vi "TestExecuteValueChangeSubscription_RejectRepeats.vi"(8 "error in (no error)":errorcluster, 11 "TestCase in":refnum<class "TestSubscriptionPolicy.lvclass">) -> (0 "error out":errorcluster, 3 "TestCase out":refnum<class "TestSubscriptionPolicy.lvclass">)   [LabVIEW 2015, in "TestSubscriptionPolicy.lvclass"]
uses:
  TestSubscriptionPolicy.lvclass
  Framework/SubscriptionPolicy/ValueChangeSubscription/ValueChangeSubscription.lvclass/ValueChangeSubscription.ctl
  Framework/SubscriptionPolicy/ValueChangeSubscription/ValueChangeSubscription.lvclass
  Framework/Transport/QueueTransport/QueueTransport.lvclass
  Framework/IMediator/ISubscriptionPolicy/ISubscriptionPolicy.lvclass
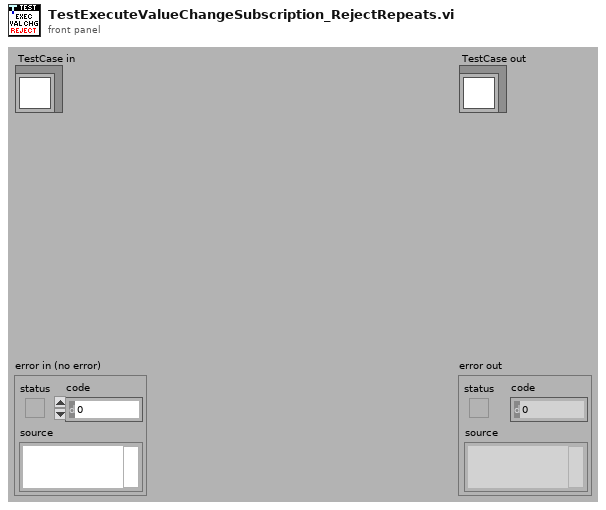
[diagram p1: front panel]
types:
  T1 = cluster{"Data":variant, "Publication Time":timestamp}
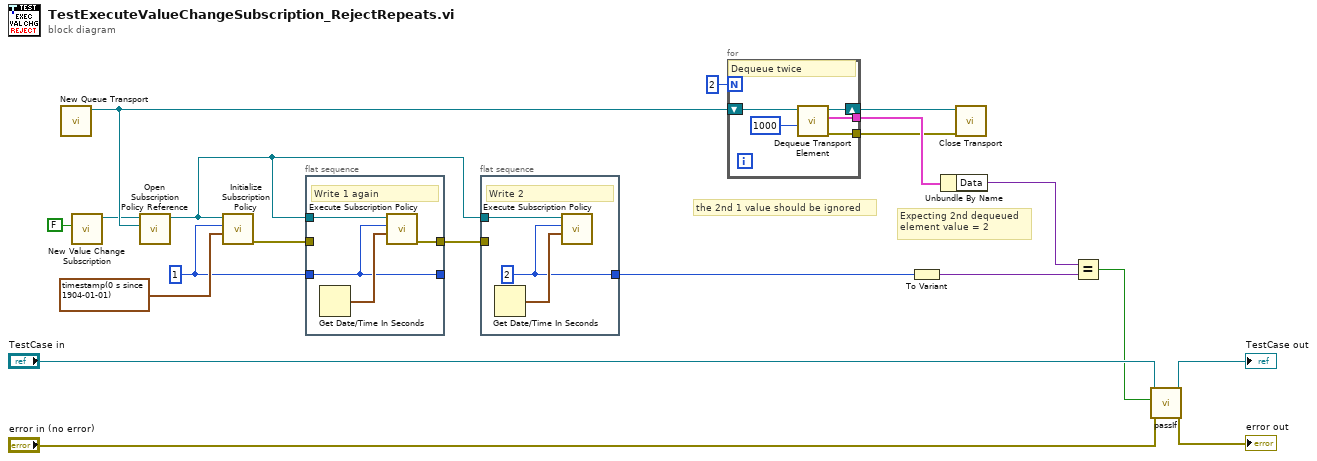
[diagram p0: block diagram]
diagram:
  w7 = 1
  # "the 2nd 1 value should be ignored"
  # "Expecting 2nd dequeued\nelement value = 2"
  n1 = call "New Queue Transport.vi"() -> ("QueueTransport Out"=w16:refnum<class "QueueTransport.lvclass">)  [unwired: 10 in, 1 out]
  n2 = call "New Value Change Subscription.vi"("Ignore Past Updates? (F)"=FALSE) -> ("ValueChangeSubscription Out"=w12:refnum<class "ValueChangeSubscription.lvclass">)  [unwired: 10 in]
  n3 = call "Open Subscription Policy Reference.vi"("Transport"=w16, "SubscriptionPolicy"=w12) -> ("Subscription Policy"=w4:refnum<data-value>)  [unwired: 8 in, 1 out]
  n4 = call "Initialize Subscription Policy.vi"("Last Publish Time"=timestamp(0 s since 1904-01-01), "Last Topic Value"=w7, "Subscription Policy"=w4) -> ("Error Out (Do Not Subscribe?)"=w5:errorcluster)  [unwired: 8 in]
  n5 = flat-sequence {
    tunnel: w7 -> [w22]
    tunnel: w4 -> [w23]
    tunnel: w5 -> [_]
    tunnel: [w22] -> _
    tunnel: [w21] -> w1
    frame #0 {
      # "Write 1 again"
      n6 = Get Date/Time In Seconds() -> (seconds since 1Jan1904=w24:timestamp)
      n7 = call "Execute Subscription Policy.vi"("Publish Time"=w24, "New Topic Value"=w22, "Subscription Policy"=w23) -> ("error out (Unsubscribe?)"=w21:errorcluster)  [unwired: 8 in]
    }
  }
  n8 = flat-sequence {
    tunnel: w4 -> [w26]
    tunnel: [w25] -> w3
    tunnel: w1 -> [_]
    frame #0 {
      w25 = 2
      # "Write 2"
      n9 = Get Date/Time In Seconds() -> (seconds since 1Jan1904=w27:timestamp)
      n10 = call "Execute Subscription Policy.vi"("Publish Time"=w27, "New Topic Value"=w25, "Subscription Policy"=w26) -> ()  [unwired: 8 in, 1 out]
    }
  }
  n11 = for {
    N: 2 -> [_]
    tunnel: [w30] -> w15
    tunnel: [w28] -> w13
    shift-right: [w29] -> w14
    shift-left: w16 -> [w32]
    # "Dequeue twice"
    n12 = call "Dequeue Transport Element.vi"("Timeout In ms (-1)"=1000, "QueueTransport in"=w32) -> ("error out"=w28:errorcluster, "Element"=w30:T1, "QueueTransport out"=w29:refnum<class "QueueTransport.lvclass">)  [unwired: 6 in, 1 out]
  }
  n13 = To Variant(anything=w3) -> (Variant=w9:variant)
  n14 = Unbundle By Name(w15) -> ("Data"=w10:variant)
  n15 = call-dynamic "Close Transport.vi"("error in (no error)"=w13, "QueueTransport in"=w14) -> ()  [unwired: 9 in, 1 out]
  n16 = Equal?(x=w10, y=w9) -> (x = y?=w6:bool)
  n17 = call-dynamic "passIf.vi"("error in (no error)"="error in (no error)", "pass"=w6, "TestCase in"="TestCase in") -> ("error out"=→"error out":errorcluster, "TestCase out"=→"TestCase out":refnum<class "TestSubscriptionPolicy.lvclass">)  [unwired: 7 in]
